vi "AreaScan3DGraph.vi"(0 "Area Scan Data":dbl[][][](array[numeric]), 1 "Area Scan Data page":i32) -> ()   [LabVIEW 2014]
doc: "3D plot of X,Y,Z data.\n\nThis VI was designed for reentrant execution and allows a visualization of area scan routine data."
uses:
  <vilib>/Native 3D Graph/xcontrol/3DPC_SurfacePlot.xctl
panel:
  in  "View Direction":T1(ring)=enum."User Define"
  in  "Graph Colors":u32[](array[colorbox])
  in  "Axes names":string[](array[string])=["X", "Y", "Z"]
  in  "Update Data":i32
  in  "stop":bool
  in  "YZ Projection":bool
  in  "XZ Projection":bool
  in  "XY Projection":bool
  in  "Scan range":T2={"Scan name"="", "Scan range minimum"=0.0, "Scan range maximum"=100.0, "Step range minimum"=0.0, "Step range maximum"=100.0}
  out "3D Graph":refnum<class "Base Datatype.lvclass">[](xcontrol)
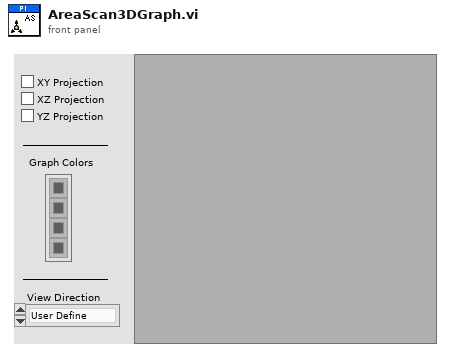
[diagram p1: front panel]
types:
  T1 = enum32{"Towards X-Y Plane", "Towards Y-Z Plane", "Towards X-Z Plane", "User Define"}
  T2 = cluster{"Scan name":string, "Scan range minimum":dbl, "Scan range maximum":dbl, "Step range minimum":dbl, "Step range maximum":dbl}
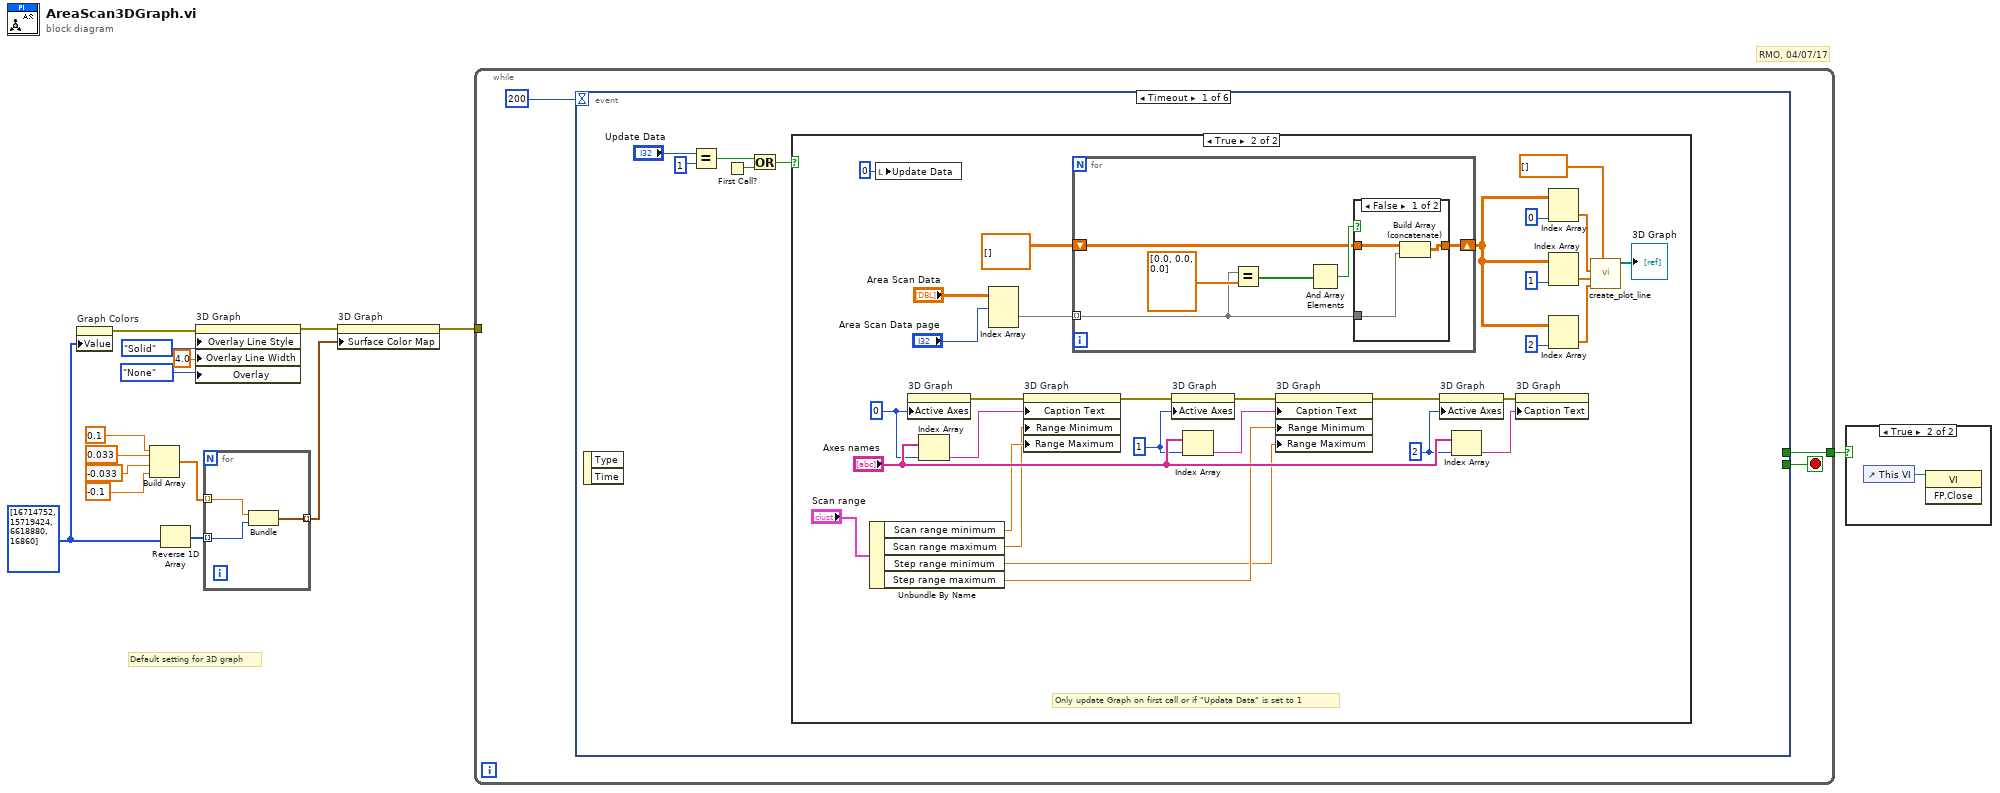
[diagram p0: block diagram]
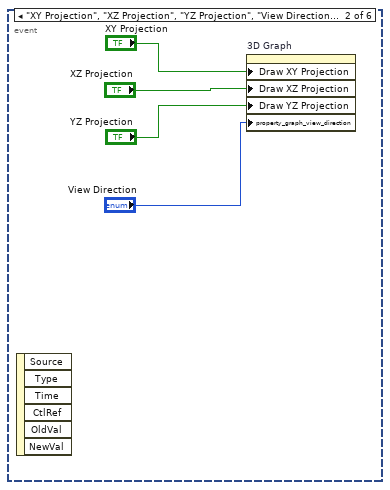
[diagram p5: hidden frame]
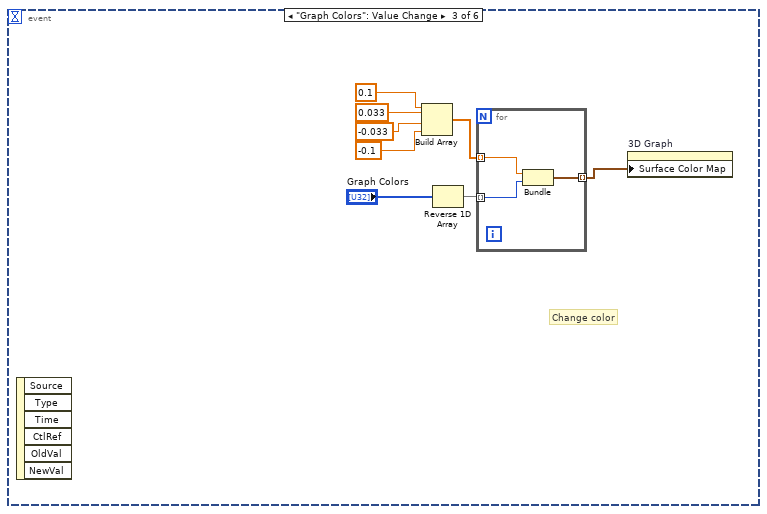
[diagram p6: hidden frame]
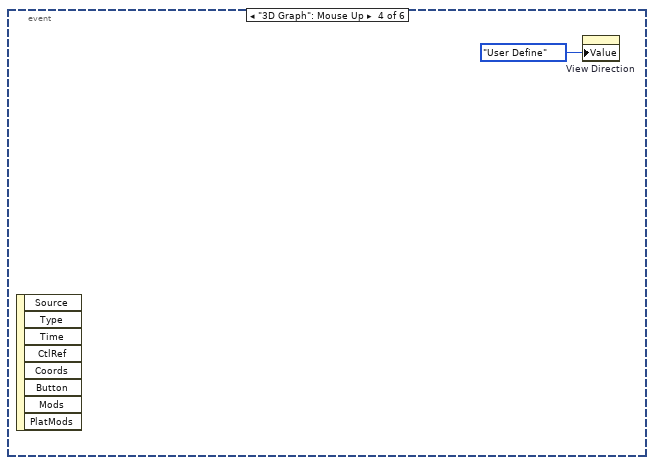
[diagram p7: hidden frame]
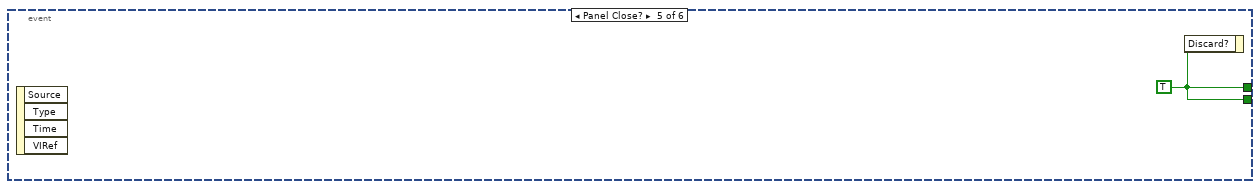
[diagram p8: hidden frame]
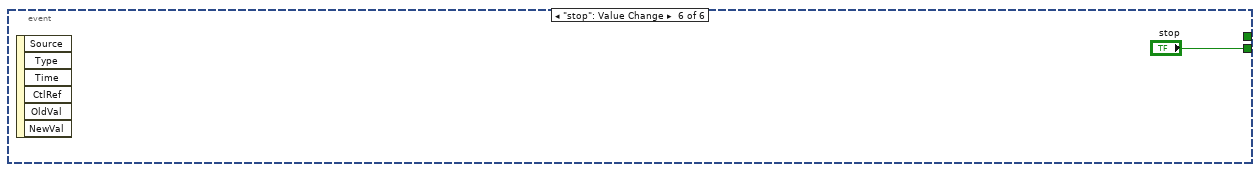
[diagram p9: hidden frame]
diagram:
  w2 = u32[] [16714752, 15719424, 6618880, 16860] ("Graph Colors")
  # "RMO, 04/07/17"
  # "Default setting for 3D graph"
  n1 = property on="Graph Colors" class="Arr (strict)"("Value"=w2) -> (error out=w1:errorcluster)  [unwired: 2 in, 1 out]
  n2 = Build Array(0.1, 0.033, -0.033, -0.1) -> (w12:dbl[])
  n3 = Reverse 1D Array(array=w2) -> (reversed array=w14:u32[])
  n4 = property on="3D Graph" class="LabVIEW 3D Graph (strict)"(error in=w1, "Overlay Line Style"=enum16{"Solid", "Dash", "Dot", "Dash Dot"}."Solid" ("Plots:Overlay Line Style"), "Overlay Line Width"=sgl 4.0 ("Plots:Overlay Line Width"), "Overlay"=enum16{"None", "Points", "Lines", "Both"}."None" ("Plots:Overlay")) -> (error out=w3:errorcluster)  [unwired: 1 in, 1 out]
  n5 = for {
    tunnel: w14 -> [w17] mode=indexing
    tunnel: w12 -> [w18] mode=indexing
    tunnel: [w16] -> w13 mode=indexing
    n6 = Bundle(w18, "Color Box"=w17) -> (w16:cluster{dbl, "Color Box":u32})  [unwired: 1 out]
  }
  n7 = property on="3D Graph" class="LabVIEW 3D Graph (strict)"(error in=w3, "Surface Color Map"=w13) -> (error out=w7:errorcluster)  [unwired: 1 in, 1 out]
  n8 = while {
    tunnel: [w19] -> w15
    tunnel: w7 -> [_]
    stop <- w21 stop-if-true
    n9 = event shown="[0] Timeout" {
      selector: _ -> [_ _ _ _ _ _]
      dyn-events: _ -> [_ _ _ _ _ _]
      timeout: 200 -> [_ _ _ _ _ _]
      tunnel: [_ _ _ _ w84 "stop"] -> w21
      tunnel: [_ _ _ _ w84 _] -> w19
      event Timeout {
        n10 = event-data() -> ()  [unwired: 3 out]
        n11 = Equal?(x="Update Data", y=1) -> (x = y?=w24:bool)
        n12 = First Call?() -> (First Call?: T/F=w23:bool)
        n13 = Or(x=w24, y=w23) -> (x .or. y?=w22:bool)
        n14 = case shown="True" w22 {
          frame False {
          }
          frame True {
            w35 = 2 ("Axes:Active Axis")
            w36 = 1 ("Axes:Active Axis")
            w37 = 0 ("Axes:Active Axis")
            # "Only update Graph on first call or if \"Updata Data\" is set to 1"
            n15 = Unbundle By Name("Scan range") -> ("Scan range minimum"=w30:dbl, "Scan range maximum"=w29:dbl, "Step range minimum"=w27:dbl, "Step range maximum"=w28:dbl)
            n16 = local write "Update Data"(0) -> ()
            n17 = property on="3D Graph" class="LabVIEW 3D Graph (strict)"("Active Axes"=w37) -> (error out=w44:errorcluster)  [unwired: 2 in, 1 out]
            n18 = Index Array(array="Axes names", index=w37) -> (element=w41:string)
            n19 = Index Array(array="Area Scan Data", index (dim 0)="Area Scan Data page") -> (element=w51:dbl[][])  [unwired: 2 in]
            n20 = property on="3D Graph" class="LabVIEW 3D Graph (strict)"(error in=w44, "Caption Text"=w41, "Range Minimum"=w29, "Range Maximum"=w30) -> (error out=w33:errorcluster)  [unwired: 1 in, 1 out]
            n21 = for {
              tunnel: w51 -> [w60] mode=indexing
              shift-right: [w58] -> w49
              shift-left: dbl[][] [] ("subarray") -> [w59]
              n22 = Equal?(x=w60, y=dbl[] [0.0, 0.0, 0.0]) -> (x = y?=w61:bool[])
              n23 = And Array Elements(Boolean array=w61) -> (logical AND=w62:bool)
              n24 = case shown="False" w62 {
                tunnel: w60 -> [w65 _]
                tunnel: w59 -> [w66 w67]
                tunnel: [w64 w67] -> w58
                frame False {
                  n25 = Build Array (concatenate)(w66, w65) -> (w64:dbl[][])
                }
                frame True {
                }
              }
            }
            n26 = property on="3D Graph" class="LabVIEW 3D Graph (strict)"(error in=w33, "Active Axes"=w36) -> (error out=w43:errorcluster)  [unwired: 1 in, 1 out]
            n27 = Index Array(array="Axes names", index=w36) -> (element=w39:string)
            n28 = property on="3D Graph" class="LabVIEW 3D Graph (strict)"(error in=w43, "Caption Text"=w39, "Range Minimum"=w28, "Range Maximum"=w27) -> (error out=w32:errorcluster)  [unwired: 1 in, 1 out]
            n29 = property on="3D Graph" class="LabVIEW 3D Graph (strict)"(error in=w32, "Active Axes"=w35) -> (error out=w42:errorcluster)  [unwired: 1 in, 1 out]
            n30 = Index Array(array="Axes names", index=w35) -> (element=w38:string)
            n31 = property on="3D Graph" class="LabVIEW 3D Graph (strict)"(error in=w42, "Caption Text"=w38) -> ()  [unwired: 1 in, 2 out]
            n32 = Index Array(array=w49, index (col)=0) -> (element=w47:dbl[])  [unwired: 1 in]
            n33 = Index Array(array=w49, index (col)=1) -> (element=w46:dbl[])  [unwired: 1 in]
            n34 = Index Array(array=w49, index (col)=2) -> (element=w48:dbl[])  [unwired: 1 in]
            n35 = call <vilib>:"create_plot_line.vi"("color vector"=dbl[] [], "z vector"=w48, "y vector"=w46, "x vector"=w47) -> ("plots out"=→"3D Graph":refnum<class "Base Datatype.lvclass">[])  [unwired: 2 in, 5 out]
          }
        }
      }
      event "XY Projection", "XZ Projection", "YZ Projection", "View Direction": Value Change {
        n36 = event-data() -> ()  [unwired: 7 out]
        n37 = property on="3D Graph" class="LabVIEW 3D Graph (strict)"("Draw XY Projection"="XY Projection", "Draw XZ Projection"="XZ Projection", "Draw YZ Projection"="YZ Projection", "property_graph_view_direction"="View Direction") -> ()  [unwired: 2 in, 2 out]
      }
      event "Graph Colors": Value Change {
        # "Change color"
        n38 = event-data() -> ()  [unwired: 7 out]
        n39 = Build Array(0.1, 0.033, -0.033, -0.1) -> (w75:dbl[])
        n40 = Reverse 1D Array(array="Graph Colors") -> (reversed array=w73:u32[])
        n41 = for {
          tunnel: w73 -> [w81] mode=indexing
          tunnel: w75 -> [w82] mode=indexing
          tunnel: [w80] -> w74 mode=indexing
          n42 = Bundle(w82, "Color Box"=w81) -> (w80:cluster{dbl, "Color Box":u32})  [unwired: 1 out]
        }
        n43 = property on="3D Graph" class="LabVIEW 3D Graph (strict)"("Surface Color Map"=w74) -> ()  [unwired: 2 in, 2 out]
      }
      event "3D Graph": Mouse Up {
        n44 = event-data() -> ()  [unwired: 9 out]
        n45 = property on="View Direction" class="Enum (strict)"("Value"=T1."User Define" ("View Direction")) -> ()  [unwired: 2 in, 2 out]
      }
      event Panel Close? {
        w84 = TRUE
        n46 = event-data() -> ()  [unwired: 5 out]
        n47 = event-data("Discard?"=w84) -> ()  [unwired: 1 in, 1 out]
      }
      event "stop": Value Change {
        n48 = event-data() -> ()  [unwired: 7 out]
      }
    }
  }
  n49 = case shown="True" w15 {
    frame False {
    }
    frame True {
      n50 = control-ref of="This VI"() -> (w86:refnum<vi>)
      n51 = invoke class="VI" method="FP.Close"(reference=w86) -> ()  [unwired: 2 in, 3 out]
    }
  }
